vi "NXT Left Wall Follow B.vi"(1 "Distance array":i16[](array[numeric])=[800, 800, 800, 400, 600, 700, 800, 600, 800, 800, 800, 800, 800, 800, 800, 800]) -> (0 "ouput array":i16[](array[numeric]))   [LabVIEW 2012]
doc: "This VI takes in the array for the scanning IR sensor. It uses a single value, at -45 degrees, to follow the left sided wall. The value at 0 degrees will turn the tug to the right."
uses:
  <vilib>/NXT/Dual Mode Library/prims/insertIntoArray/insertArrayIntoArray_int.vi
panel:
  out "Degrees\nShift":sgl
  out "Distance Array":cluster{i32, i32, "Left Wall array":i16[]}(graph)
  out "Left Wall array out":cluster{i32, i32, "ouput array":i32[]}(graph)
  out "Shift":i32
  out "Left Wall array":cluster{i32, i32, "Left Wall array":i16[]}(graph)
  # "This routine expects the IR sensor to scan between index values of 3 and 7...the other will all have the value of 800\nThe index 3 represents an angle of 50 degrees to port of the tug.\nThe index of 7 represents an angle of 5.6 degrees to port of the tug.\n\nThe routine tries to keep a distance of between 425mm and 675mm from the wall measured at 50 degrees.\nUsing the value at index 3 alone, this is about 450mm normal to the wall.\n\nIf the index 7 has a value below 750...the tug will turn right."
  # "3"
  # "7"
  # "8"
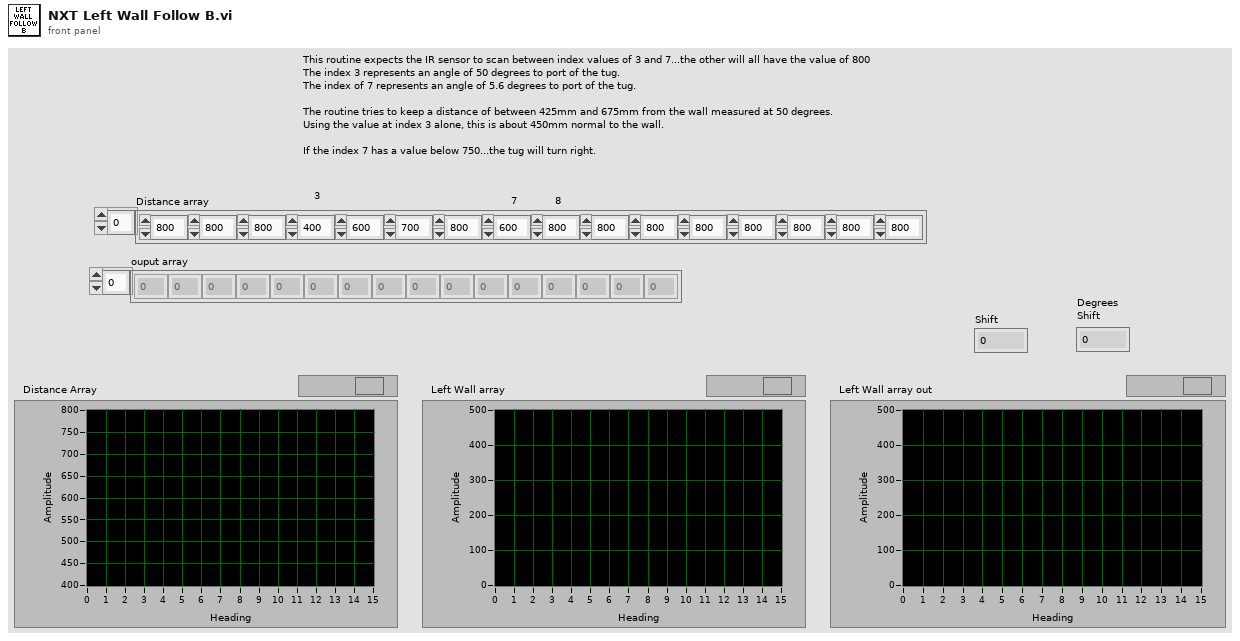
[diagram p1: front panel]
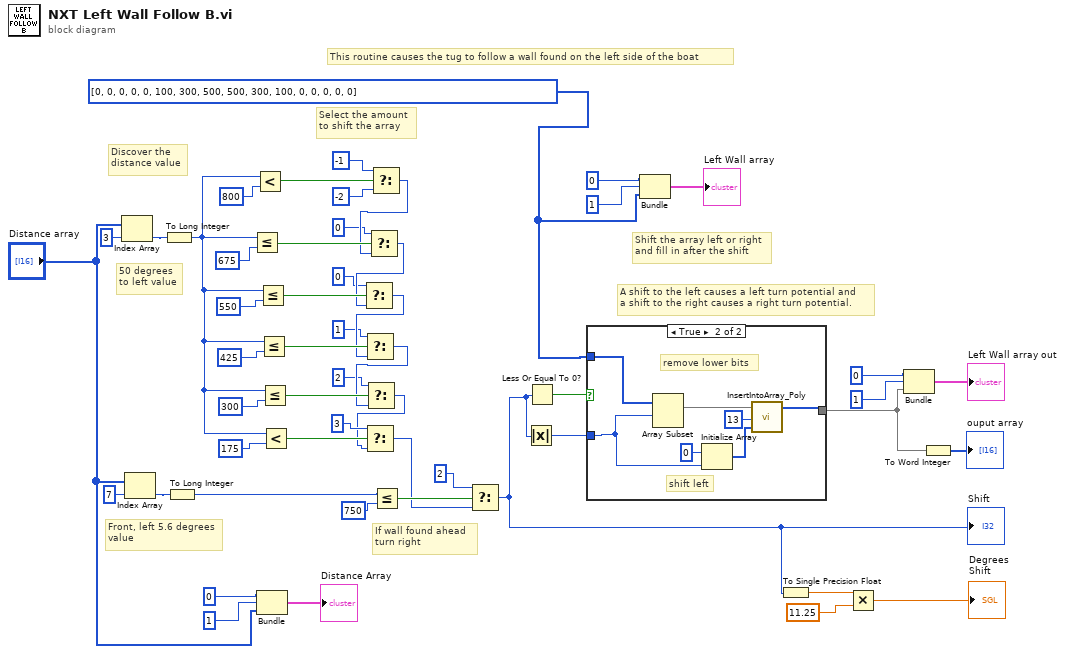
[diagram p0: block diagram]
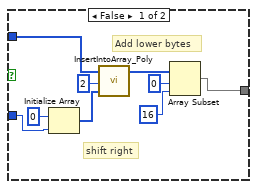
[diagram p2: hidden frame]
diagram:
  w21 = i16[] [0, 0, 0, 0, 0, 100, 300, 500, 500, 300, 100, 0, 0, 0, 0, 0] ("Left Wall array")
  # "50 degrees\nto left value"
  # "Front, left 5.6 degrees\nvalue"
  # "If wall found ahead\nturn right"
  # "A shift to the left causes a left turn potential and\na shift to the right causes a right turn potential."
  # "This routine causes the tug to follow a wall found on the left side of the boat"
  # "Shift the array left or right\nand fill in after the shift"
  # "Select the amount\nto shift the array"
  # "Discover the\ndistance value"
  n1 = Index Array(array="Distance array", index=3) -> (element=w13:i16)
  n2 = Index Array(array="Distance array", index=7) -> (element=w11:i16)
  n3 = To Long Integer(number=w13) -> (32bit integer=w14:i32)
  n4 = To Long Integer(number=w11) -> (32bit integer=w10:i32)
  n5 = Less Or Equal?(x=w14, y=675) -> (x <= y?=w45:bool)
  n6 = Less?(x=w14, y=800) -> (x < y?=w49:bool)
  n7 = Bundle(0, 1, "Distance array"="Distance array") -> (→"Distance Array":cluster{i32, i32, "Distance array":i16[]})  [unwired: 1 in]
  n8 = Less Or Equal?(x=w14, y=550) -> (x <= y?=w43:bool)
  n9 = Less Or Equal?(x=w14, y=425) -> (x <= y?=w41:bool)
  n10 = Less Or Equal?(x=w14, y=300) -> (x <= y?=w39:bool)
  n11 = Less?(x=w14, y=175) -> (x < y?=w20:bool)
  n12 = Select(t=-1, s=w49, f=-2) -> (s? t:f=w36:i32)
  n13 = Select(t=0, s=w45, f=w36) -> (s? t:f=w35:i32)
  n14 = Select(t=0 ("f"), s=w43, f=w35) -> (s? t:f=w34:i32)
  n15 = Select(t=1 ("f"), s=w41, f=w34) -> (s? t:f=w33:i32)
  n16 = Select(t=2 ("f"), s=w39, f=w33) -> (s? t:f=w18:i32)
  n17 = Select(t=3, s=w20, f=w18) -> (s? t:f=w16:i32)
  n18 = Less Or Equal?(x=w10, y=750) -> (x <= y?=w22:bool)
  n19 = Select(t=2 ("f"), s=w22, f=w16) -> (s? t:f=w3:i32)
  "Shift" <- w3
  n20 = Absolute Value(x=w3) -> (abs(x)=w37:i32)
  n21 = Less Or Equal To 0?(x=w3) -> (x <= 0?=w38:bool)
  n22 = case shown="True" w38 {
    tunnel: w37 -> [w59 w64]
    tunnel: w21 -> [w62 w69]
    tunnel: [w56 w63] -> w25
    frame False {
      # "shift right"
      # "Add lower bytes"
      n23 = Initialize Array(0 ("element"), w59) -> (w58:i32[])
      n24 = call-poly <vilib>:"InsertIntoArray_Poly.vi"("array"=w62, "index"=2, "element or subarray"=w58) -> ("ouput array"=w57:i32[])  [unwired: 24 in]
      n25 = Array Subset(array=w57, index=0, length=16) -> (w56:i32[])
    }
    frame True {
      # "shift left"
      # "remove lower bits"
      n26 = Array Subset(array=w69, index=w64) -> (w65:i16[])  [unwired: 1 in]
      n27 = Initialize Array(0 ("element"), w64) -> (w68:i32[])
      n28 = call-poly <vilib>:"InsertIntoArray_Poly.vi"("array"=w65, "index"=13, "element or subarray"=w68) -> ("ouput array"=w63:i32[])  [unwired: 24 in]
    }
  }
  n29 = Bundle(0, 1, "Left Wall array"=w21) -> (→"Left Wall array":cluster{i32, i32, "Left Wall array":i16[]})  [unwired: 1 in]
  n30 = To Single Precision Float(number=w3) -> (single precision float=w2:sgl)
  n31 = Multiply(x=w2, y=sgl 11.25) -> (x*y=→"Degrees\nShift":sgl)
  n32 = Bundle(0, 1, "ouput array"=w25) -> (→"Left Wall array out":cluster{i32, i32, "ouput array":i32[]})  [unwired: 1 in]
  n33 = To Word Integer(number=w25) -> (16bit integer=→"ouput array":i16[])
